vi "Open Config Data.vi"(8 "error in (no error)":errorcluster, 10 "create file if necessary (T)":bool=TRUE, 11 "configuration file path":path) -> (0 "error out":errorcluster, 2 "file created?":bool, 3 "refnum":T1)   [LabVIEW 2020, in "NI_LVConfig.lvlib"]
doc: "Opens a reference to the configuration data found in a platform-independent configuration file."
uses:
  <vilib>/Utility/config.llb/NI_LVConfig.lvlib
  <vilib>/Utility/config.llb/Config Data RefNum.ctl
  <vilib>/Utility/config.llb/Config Data.ctl
  <vilib>/Utility/config.llb/Section.ctl
  <vilib>/Utility/config.llb/8.6CompatibleGlobalVar.vi
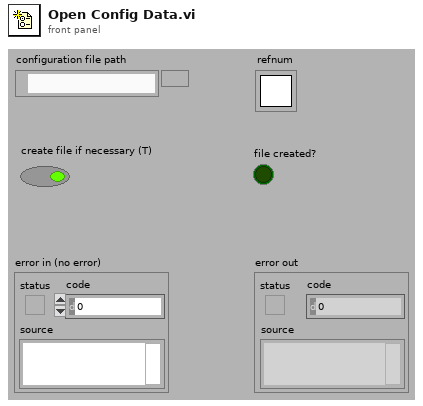
[diagram p1: front panel]
types:
  T1 = typedef "NI_LVConfig.lvlib/Config Data RefNum.ctl" = refnum<k1>
  T2 = typedef "NI_LVConfig.lvlib/Config Data.ctl" = cluster{"sections":T3[], "path":path, "dirty":bool}
  T3 = typedef "NI_LVConfig.lvlib/Section.ctl" = cluster{"name":string, "comment":string, "kvc":string[][]}
  T4 = typedef "NI_LVConfig.lvlib/Config Queue.ctl" = refnum<queue>
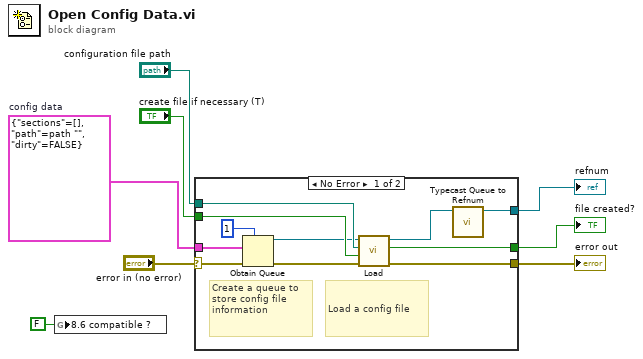
[diagram p0: block diagram]
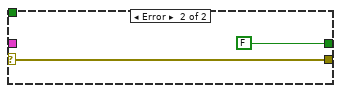
[diagram p2: hidden frame]
diagram:
  w2 = T2 {"sections"=[], "path"=path "", "dirty"=FALSE}  # config data
  n1 = global write "8.6CompatibleGlobalVar.vi" "8.6 compatible ?"(FALSE ("8.6 compatible ?")) -> ()
  n2 = case shown="No Error" "error in (no error)" {
    selector: "error in (no error)" -> [w14 w21]
    tunnel: "configuration file path" -> [w19 _]
    tunnel: "create file if necessary (T)" -> [w18 _]
    tunnel: [w16 FALSE ("file created?")] -> w4
    tunnel: [w17 w21] -> w5
    tunnel: w2 -> [w13 _]
    tunnel: [w10 _] -> w3
    frame No Error {
      # "Load a config file"
      # "Create a queue to store config file information"
      n3 = Obtain Queue(max queue size (-1, unlimited)=1, element data type=w13, error in (no error)=w14) -> (queue out=w9:refnum<queue>, error out=w12:errorcluster)  [unwired: 2 in, 1 out]
      n4 = call <vilib>:"Load.vi"("error in (no error)"=w12, "create file if necessary? (T)"=w18, "configuration file path"=w19, "queue in"=w9) -> ("error out"=w17:errorcluster, "file created?"=w16:bool, "queue out"=w11:T4)  [unwired: 1 in, 4 out]
      n5 = call <vilib>:"Typecast Queue to Refnum.vi"("queue in"=w11) -> ("refnum out"=w10:T1)  [unwired: 10 in]
    }
    frame Error {
    }
  }
  "error out" <- w5
  "file created?" <- w4
  "refnum" <- w3
